vi "ineter cycle delay.vi"(10 "urge":u8, 11 "array in":i16[](array[numeric])=[0, 0, 0, 0, 0, 0, 0, 0, 0, 0, 0, 0, 0, 0, 0, 0]) -> (3 "delayed data":i16[](array[numeric]))   [LabVIEW 2021]
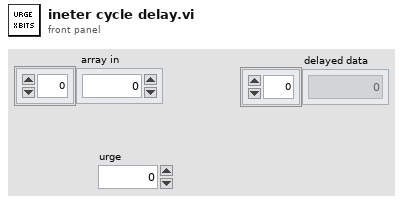
[diagram p1: front panel]
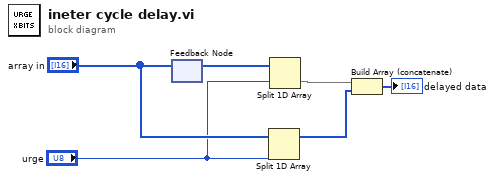
[diagram p0: block diagram]
diagram:
  n1 = feedback-in #1("array in") -> ()
  n2 = feedback #1() -> (w6:i16[])  [unwired: 1 in]
  n3 = Split 1D Array(array="array in", index="urge") -> (first subarray=w3:i16[])  [unwired: 1 out]
  n4 = Split 1D Array(array=w6, index="urge") -> (second subarray=w4:i16[])  [unwired: 1 out]
  n5 = Build Array (concatenate)(w4, w3) -> (→"delayed data":i16[])
